vi "UniRecAll.vi"() -> ()   [LabVIEW 2011]
uses:
  <instrlib>/niHWS/nihws.llb/niHWS Open File Permissions ID.ctl
  <vilib>/DAQmx/read.llb/DAQmx Read (Analog 1D Wfm NChan NSamp).vi
  <vilib>/DAQmx/create/channels.llb/DAQmx Create Channel (AI-Voltage-Basic).vi
  <vilib>/DAQmx/configure/timing.llb/DAQmx Timing (Sample Clock).vi
  <instrlib>/niHWS/nihws.llb/niHWS Write Analog DBL.vi
  <vilib>/DAQmx/miscellaneous.llb/DAQmx Fill In Error Info.vi
  <instrlib>/niHWS/nihws.llb/niHWS Write Analog WDT.vi
  <vilib>/gmath/NI_Gmath.lvlib
  C:/Program Files/National Instruments/LabVIEW 2011/resource/objmgr/daqmx.rc
panel:
  in  "Recording channels":tag="4498_1/ai1, 4498_1/ai3, 4498_1/ai5, 4498_1/ai7"
  in  "Recording Path":path
  out "File":bool
  in  "stop":bool
  in  "Record":bool
  in  "Offset":dbl=0.0001
  out "Waveform Chart 2":waveform(dbl)[](graph)
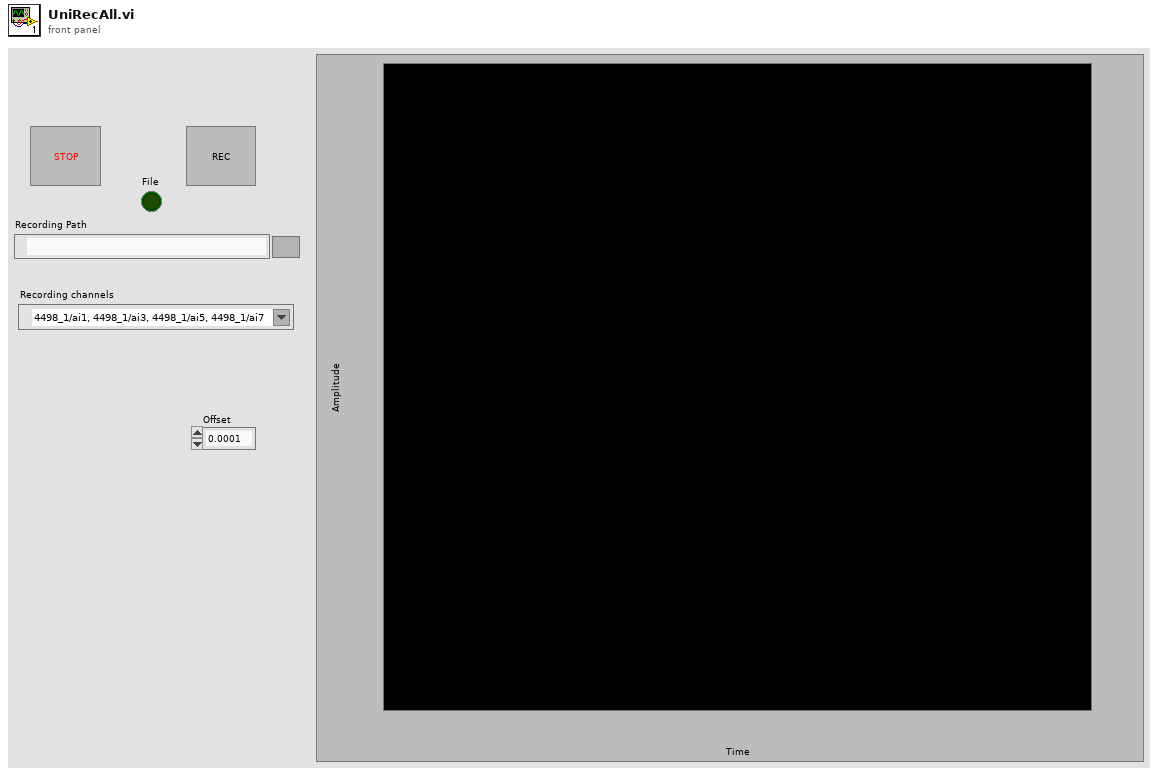
[diagram p1: front panel]
types:
  T1 = typedef "niHWS Open File Permissions ID.ctl" = enum32{"Read Only", "Read/Write Existing", "Read/Write/Create New", "Read/Write/Create New Always"}
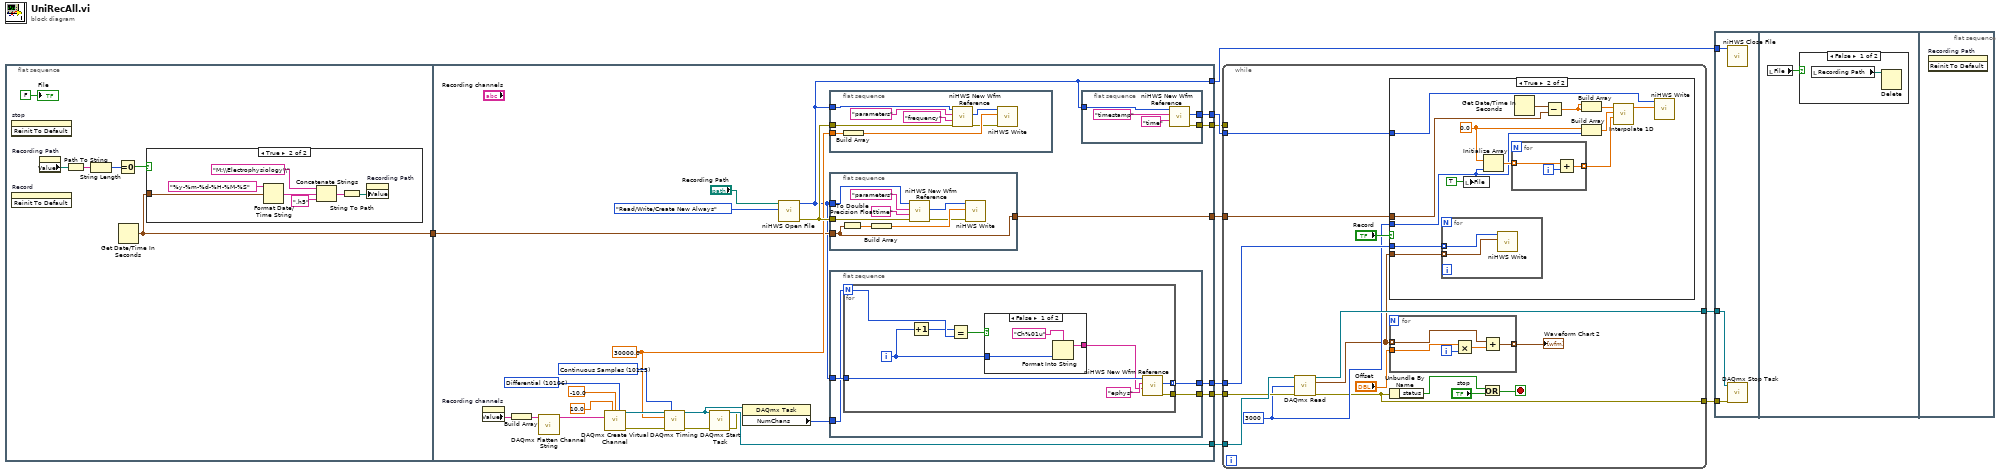
[diagram p0: block diagram]
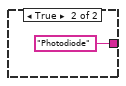
[diagram p4: hidden frame]
diagram:
  n1 = flat-sequence {
    tunnel: [w12] -> w10
    tunnel: [w48] -> w9
    tunnel: [w47] -> w8
    tunnel: [w46] -> w7
    tunnel: [w45] -> w4
    tunnel: [w44] -> w3
    tunnel: [w43] -> w2
    tunnel: w10 -> [w26]
    tunnel: [w25] -> w1
    frame #0 {
      n2 = invoke on="stop" class="Bool (strict)" method="Reinit To Default"() -> ()  [unwired: 3 in, 3 out]
      n3 = invoke on="Record" class="Bool (strict)" method="Reinit To Default"() -> ()  [unwired: 3 in, 3 out]
      n4 = property on="Recording Path" class="Path"() -> ("Value"=w13:path)  [unwired: 2 in, 2 out]
      n5 = Path To String(path=w13) -> (string=w14:string)
      n6 = String Length(string=w14) -> (length=w15:i32)
      n7 = Equal To 0?(x=w15) -> (x = 0?=w16:bool)
      n8 = Get Date/Time In Seconds() -> (seconds since 1Jan1904=w12:timestamp)
      n9 = case shown="True" w16 {
        tunnel: w12 -> [_ w21]
        frame False {
        }
        frame True {
          n10 = Format Date/Time String(time format string (%c)="%y-%m-%d-%H-%M-%S", seconds (now)=w21) -> (date/time string=w18:string)  [unwired: 1 in]
          n11 = Concatenate Strings("M:\\Electrophysiology\\", w18, ".h5") -> (w19:string)
          n12 = String To Path(string=w19) -> (path=w23:path)
          n13 = property on="Recording Path" class="Path"("Value"=w23) -> ()  [unwired: 2 in, 2 out]
        }
      }
      "File" <- FALSE
    }
    frame #1 {
      w24 = 10106 items=["default"=-1, "RSE"=10083, "NRSE"=10078, "Differential"=10106, "Pseudodifferential"=12529] ("input terminal configuration")
      w39 = 10123 items=["Finite Samples"=10178, "Continuous Samples"=10123, "Hardware Timed Single Point"=12522] ("sample mode")
      w30 = 30000.0 ("rate")
      n14 = property on="Recording channels" class="DAQmxName"() -> ("Value"=w27:string)  [unwired: 2 in, 2 out]
      n15 = Build Array(w27) -> (w29:string[])
      n16 = call <vilib>:"DAQmx Flatten Channel String.vi"("names in"=w29) -> ("names out"=w28:string)  [unwired: 13 in, 1 out]
      n17 = call-poly <vilib>:"DAQmx Create Virtual Channel.vi"("maximum value"=10.0, "minimum value"=-10.0, "input terminal configuration"=w24, "physical channels"=w28) -> ("task out"=w40:refnum<k21>, "error out"=w38:errorcluster)  [unwired: 10 in]
      n18 = call-poly <vilib>:"DAQmx Timing.vi"("task/channels in"=w40, "sample mode"=w39, "rate"=w30, "error in"=w38) -> ("task out"=w35:refnum<k21>, "error out"=w37:errorcluster)  [unwired: 10 in]
      n19 = call <vilib>:"DAQmx Start Task.vi"("task/channels in"=w35, "error in"=w37) -> ("task out"=w48:refnum<k21>, "error out"=w36:errorcluster)  [unwired: 12 in]
      n20 = property class="DAQmx Task"(reference=w35, error in=w36) -> ("NumChans"=w31:u32)  [unwired: 2 out]
      n21 = call <instrlib>:"niHWS Open File.vi"("permissions (0:read only)"=niHWS_Open_File_Permissions_ID."Read/Write/Create New Always", "file path"="Recording Path") -> ("error out"=w32:errorcluster, "file handle"=w25:u32)  [unwired: 8 in]
      n22 = flat-sequence {
        tunnel: w30 -> [w66]
        tunnel: w32 -> [w65]
        tunnel: w25 -> [w64]
        frame #0 {
          n23 = Build Array(w66) -> (w67:dbl[])
          n24 = call <instrlib>:"niHWS New Wfm Reference.vi"("error in (no error)"=w65, "waveform name (empty)"="frequency" ("group name (empty)"), "group name (empty)"="parameters", "file handle in"=w64) -> ("error out"=w63:errorcluster, "waveform reference"=w70:u32)  [unwired: 5 in, 1 out]
          n25 = call-poly <instrlib>:"niHWS Write.vi"("error in (no error)"=w63, "data"=w67, "waveform reference in"=w70) -> ()  [unwired: 7 in, 2 out]
        }
      }
      n26 = flat-sequence {
        tunnel: w32 -> [w62]
        tunnel: w25 -> [w61]
        tunnel: [w54] -> w43
        tunnel: w26 -> [w54]
        frame #0 {
          n27 = To Double Precision Float(number=w54) -> (double precision float=w60:dbl)
          n28 = Build Array(w60) -> (w59:dbl[])
          n29 = call <instrlib>:"niHWS New Wfm Reference.vi"("error in (no error)"=w62, "waveform name (empty)"="time" ("group name (empty)"), "group name (empty)"="parameters", "file handle in"=w61) -> ("error out"=w55:errorcluster, "waveform reference"=w56:u32)  [unwired: 5 in, 1 out]
          n30 = call-poly <instrlib>:"niHWS Write.vi"("error in (no error)"=w55, "data"=w59, "waveform reference in"=w56) -> ()  [unwired: 7 in, 2 out]
        }
      }
      n31 = flat-sequence {
        tunnel: w31 -> [w73]
        tunnel: w25 -> [w74]
        tunnel: [w72] -> w47
        tunnel: [w71] -> w46
        frame #0 {
          n32 = for {
            N: w73 -> [w78]
            tunnel: [w80] -> w72 mode=indexing
            tunnel: [w79] -> w71
            tunnel: w74 -> [w83]
            i -> [w77]
            n33 = Increment(x=w77) -> (x+1=w76:i32)
            n34 = Equal?(x=w76, y=w78) -> (x = y?=w75:bool)
            n35 = case shown="False" w75 {
              tunnel: w77 -> [w86 _]
              tunnel: [w84 "Photodiode"] -> w81
              frame False {
                n36 = Format Into String(format string="Ch%01u", w86) -> (resulting string=w84:string)  [unwired: 2 in, 1 out]
              }
              frame True {
              }
            }
            n37 = call <instrlib>:"niHWS New Wfm Reference.vi"("waveform name (empty)"=w81, "group name (empty)"="ephys", "file handle in"=w83) -> ("error out"=w79:errorcluster, "waveform reference"=w80:u32)  [unwired: 6 in, 1 out]
          }
        }
      }
      n38 = flat-sequence {
        tunnel: [w53] -> w45
        tunnel: [w52] -> w44
        tunnel: w25 -> [w50]
        frame #0 {
          n39 = call <instrlib>:"niHWS New Wfm Reference.vi"("waveform name (empty)"="time" ("format string"), "group name (empty)"="timestamp", "file handle in"=w50) -> ("error out"=w52:errorcluster, "waveform reference"=w53:u32)  [unwired: 6 in, 1 out]
        }
      }
    }
  }
  n40 = while {
    tunnel: w9 -> [w100]
    tunnel: w8 -> [w95]
    tunnel: w7 -> [w99]
    tunnel: [w98] -> w6
    tunnel: [w90] -> w5
    tunnel: w4 -> [w94]
    tunnel: w3 -> [_]
    tunnel: w2 -> [w93]
    stop <- w102 stop-if-true
    w91 = 3000 ("number of samples per channel")
    n41 = call-poly <vilib>:"DAQmx Read.vi"("task/channels in"=w100, "number of samples per channel"=w91, "error in"=w99) -> ("task out"=w98:refnum<k21>, "data"=w88:waveform(dbl)[], "error out"=w90:errorcluster)  [unwired: 10 in]
    n42 = case shown="True" "Record" {
      tunnel: w88 -> [_ w118]
      tunnel: w95 -> [_ w121]
      tunnel: w94 -> [_ w109]
      tunnel: w93 -> [_ w119]
      tunnel: w91 -> [_ w112]
      frame False {
      }
      frame True {
        w111 = 0.0 ("element")
        n43 = for {
          tunnel: w118 -> [w126] mode=indexing
          tunnel: w121 -> [w125] mode=indexing
          n44 = call-poly <instrlib>:"niHWS Write.vi"("analog waveform"=w126, "waveform reference in"=w125) -> ()  [unwired: 8 in, 2 out]
        }
        n45 = local write "File"(TRUE) -> ()
        n46 = Initialize Array(w111, w112) -> (w113:dbl[])
        n47 = for {
          tunnel: w113 -> [w124] mode=indexing
          tunnel: [w122] -> w110 mode=indexing
          i -> [w123]
          n48 = Add(x=w124, y=w123) -> (x+y=w122:dbl)
        }
        n49 = Get Date/Time In Seconds() -> (seconds since 1Jan1904=w120:timestamp)
        n50 = Subtract(x=w120, y=w119) -> (x-y=w117:dbl)
        n51 = Build Array(w117, w117) -> (w116:dbl[])
        n52 = Build Array(w111, w112) -> (w114:dbl[])
        n53 = call <vilib>:"Interpolate 1D.vi"("xi"=w110, "X"=w114, "Y"=w116) -> ("yi"=w115:dbl[])  [unwired: 6 in, 2 out]
        n54 = call-poly <instrlib>:"niHWS Write.vi"("data"=w115, "waveform reference in"=w109) -> ()  [unwired: 8 in, 2 out]
      }
    }
    n55 = for {
      tunnel: "Offset" -> [w107]
      tunnel: [w103] -> w89 mode=indexing
      tunnel: w88 -> [w105] mode=indexing
      i -> [w104]
      n56 = Multiply(x=w107, y=w104) -> (x*y=w106:dbl)
      n57 = Add(x=w105, y=w106) -> (x+y=w103:waveform(dbl))
    }
    "Waveform Chart 2" <- w89
    n58 = Unbundle By Name(w90) -> ("status"=w97:bool)
    n59 = Or(x=w97, y="stop") -> (x .or. y?=w102:bool)
  }
  n60 = flat-sequence {
    tunnel: w6 -> [w129]
    tunnel: w5 -> [w128]
    tunnel: w1 -> [w127]
    frame #0 {
      n61 = call <instrlib>:"niHWS Close File.vi"("file handle"=w127) -> ()  [unwired: 10 in, 1 out]
      n62 = call <vilib>:"DAQmx Stop Task.vi"("task/channels in"=w129, "error in"=w128) -> ()  [unwired: 12 in, 2 out]
    }
    frame #1 {
      n63 = local read "File"() -> (w130:bool)
      n64 = case shown="False" w130 {
        frame False {
          n65 = local read "Recording Path"() -> (w131:path)
          n66 = Delete(path (use dialog)=w131) -> ()  [unwired: 4 in, 3 out]
        }
        frame True {
        }
      }
    }
    frame #2 {
      n67 = invoke on="Recording Path" class="Path" method="Reinit To Default"() -> ()  [unwired: 3 in, 3 out]
    }
  }
